vi "exercise example 1.vi"(1 "x1":dbl(slide) scale=0.0..10.0, 2 "y 2":dbl, 3 "y1":dbl, 4 "x2":dbl) -> (0 "indicator":dbl)   [LabVIEW 2023]
panel:
  in  "Numeric":dbl
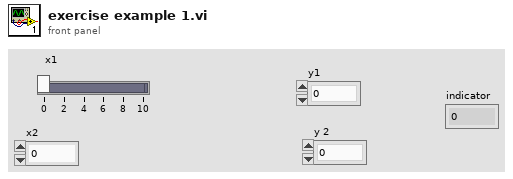
[diagram p1: front panel]
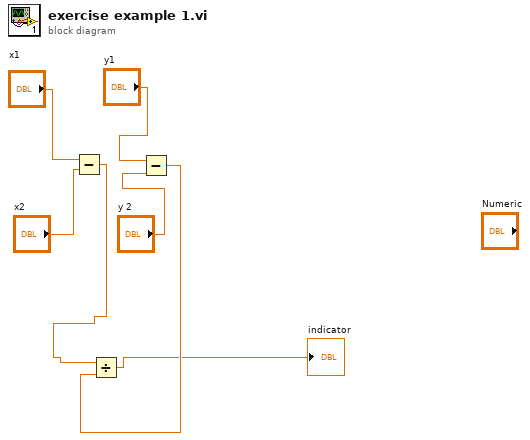
[diagram p0: block diagram]
diagram:
  n1 = Subtract(x="x1", y="x2") -> (x-y=w3:dbl)
  n2 = Subtract(x="y1", y="y 2") -> (x-y=w2:dbl)
  n3 = Divide(x=w3, y=w2) -> (x/y=→"indicator":dbl)
